vi "FPGANic-Tester.vi"() -> ()   [LabVIEW 2018]
uses:
  Source.Machine.Settings.ctl
  FPGANic.Events.ctl
  <vilib>/Field R&D Services/Logger/Private/Manager.vi
  <vilib>/FPGAPlugInAG/Dynamic/niLvFpga_Download_Dynamic.vi
  <vilib>/Utility/error.llb/Error Cluster From Error Code.vi
  <vilib>/rvi/errors/niLvFpgaAdjustHostInterfaceError.vi
  <vilib>/FPGAPlugInAG/Dynamic/niLvFpga_Run_Dynamic.vi
  FPGANic.Globals.vi
  <vilib>/FPGAPlugInAG/Dynamic/niLvFpga_Close_Dynamic.vi
  <vilib>/rvi/interface/nirviMethod/nirviMethod.xnode
  <vilib>/rvi/interface/nirviReadWriteControl/nirviReadWriteControl.xnode
  <vilib>/rvi/interface/nirviCloseFPGA/nirviCloseFPGA.xnode
  <vilib>/FPGAPlugInAG/Dynamic/niLvFpga_ReadFifo_Dynamic.vi
  <vilib>/rvi/errors/niLvFpgaMergeErrorWithErrorCode.vi
  <vilib>/FPGAPlugInAG/Dynamic/niLvFpga_WriteFifo_Dynamic.vi
  NiFpgaLv.dll
  <vilib>/rvi/interface/Simulation/niFpgaSimulationCallBeginRW.vi
  <vilib>/Field R&D Services/Logger/Logger.lvlib
panel:
  in  "Clear Debug FIFOS?":bool
  in  "Clear":bool
  in  "Read UART":bool
  in  "Tab Control":T1(tab)=enum."Configuration"
  in  "Ethernet II Params":T2={"Destination MAC"=[0, 2, 201, 85, 8, 68], "Source MAC"=[0, 1, 2, 3, 4, 5], "EtherType"=2048} {"Destination MAC" format="%.0x"; "Source MAC" format="%.02x"; "EtherType" format="%.0x"}
  in  "IPv4 Params":T3={"Destination IP"=[10, 0, 1, 100], "Source IP"=[10, 0, 1, 101], "Protocol"=17}
  in  "UDP Params":T4={"Source Port"=35312, "Destination Port"=35312, "Payload"="ABCD"}
  in  "MAC & IP":T5={"MAC Address"=[0, 1, 2, 3, 4, 5], "IP Address"=[10, 0, 1, 101]} {"MAC Address" format="%.0x"}
  out "Write Probe 2":u64[](array[numeric]) format="%.0x"
  out "Write Probe 1":u64[](array[numeric]) format="%.0x"
  out "Read Probe":u64[](array[numeric])=[11817445486661492224, 11817446517453291522, 11817445490022484036, 11817446517571077376, 11817445486650471966, 11817446518510649105, 11817445488139373056, 11817446517460230144, 11817445486661145833, 11817446517787656260, 11817445487417098240, 11817446519651434496, 11817445486644756480, 11817446517436909932, 11817445488513474924, 11817446519188976500, 11817445486735683427, 11817446519071309824, 11817445486669857024, 11817446517436872704, 11817445486712455169, 11817446519127149568, 11817445487441608960, 11817446517436872704, 11817445486741163008, 11817445692824123692, 11817726961621401602, 11817445490939658239, 11817446521731743746, 11817445490022484036, 11817446517571452929, 11817445486778910212, 11817446517436907522, 11817445490022484036, 11817446517604614500, 11817445486644690944, 11817446517436880915, 11817445488902144000, 11817446517436841984, 11817445486644690944, 11817446517436841984, 11817445486644690944, 11817445488835018955, 11817726961621401602, 11817445490939658239, 11817446521731743746, 11817445490022484036, 11817446517571452929, 11817445486778910212, 11817446517436907522, 11817445490022484036, 11817446517604614500, 11817445486644690944, 11817446517436895620, 11817445489682350080, 11817446517436841984, 11817445486644690944, 11817446517436841984, 11817445486644690944, 11817445488759354791, 11817726961621401602, 11817445490939658239, 11817446521731743746, 11817445490022484036, 11817446517571452929, 11817445486778910212, 11817446517436907522, 11817445490022484036, 11817446517604614500, 11817445486644690944, 11817446517436880915, 11817445488902144000, 11817446517436841984, 11817445486644690944, 11817446517436841984, 11817445486644690944, 11817445488835018955, 11817726961621401602, 11817445490939658239, 11817446521731743746, 11817445490022484036, 11817446517571452929, 11817445486778910212, 11817446517436907522, 11817445490022484036, 11817446517604614500, 11817445486644690944, 11817446517436878035, 11817445489493540864, 11817446517436841984, 11817445486644690944, 11817446517436841984, 11817445486644690944, 11817445489115705299, 11817726961621401602, 11817445490939658239, 11817446521731743746, 11817445490022484036, 11817446517571452929, 11817445486778910212, 11817446517436907522, 11817445490022484036, 11817446517604614500, 11817445486644690944, 11817446517436880915, 11817445488902144000, 11817446517436841984, 11817445486644690944, 11817446517436841984, 11817445486644690944, 11817445488835018955, 11817726961621401602, 11817445490939658239, 11817446521731743746, 11817445490022484036, 11817446517571452929, 11817445486778910212, 11817446517436907522, 11817445490022484036, 11817446517604614500, 11817445486644690944, 11817446517436878035, 11817445489493540864, 11817446517436841984, 11817445486644690944, 11817446517436841984, 11817445486644690944, 11817445489115705299, 11817726961621401602, 11817445490939658239, 11817446521731743746, 11817445490022484036, 11817446517571452929, 11817445486778910212, 11817446517436907522, 11817445490022484036, 11817446517604614500, 11817445486644690944, 11817446517436878035, 11817445489493540864, 11817446517436841984, 11817445486644690944, 11817446517436841984, 11817445486644690944, 11817445489115705299, 11817726961621401602, 11817445490939658239, 11817446521731743746, 11817445490022484036, 11817446517571452929, 11817445486778910212, 11817446517436907522, 11817445490022484036, 11817446517604614500, 11817445486644690944, 11817446517436880915, 11817445488902144000, 11817446517436841984, 11817445486644690944, 11817446517436841984, 11817445486644690944, 11817445488835018955, 11817726961621401602, 11817445486661492224, 11817446517453291522, 11817445490022484036, 11817446517571077376, 11817445486650474301, 11817446518510649105, 11817445487986346496, 11817446517460230144, 11817445486661145833, 11817446517787656260, 11817445487417098240, 11817446519651434496, 11817445486644756480, 11817446517436909932, 11817445488513474924, 11817446519188976500, 11817445486735683427, 11817446519071309824, 11817445486669857024, 11817446517436872704, 11817445486712455169, 11817446519127149568, 11817445487441608960, 11817446517436872704, 11817445486741163008, 11817445692824141017, 11817726961621401602, 11817445490939658239, 11817446521731743746, 11817445490022484036, 11817446517571452929, 11817445486778910212, 11817446517436907522, 11817445490022484036, 11817446517604614500, 11817445486644690944, 11817446517436878035, 11817445489493540864, 11817446517436841984, 11817445486644690944, 11817446517436841984, 11817445486644690944, 11817445489115705299, 11817726961621401602, 11817445490939658239, 11817446521731743746, 11817445490022484036, 11817446517571452929, 11817445486778910212, 11817446517436907522, 11817445490022484036, 11817446517604614500, 11817445486644690944, 11817446517436859339, 11817445486682636288, 11817446517436841984, 11817445486644690944, 11817446517436841984, 11817445486644690944, 11817445488555902218, 11817726961621401602, 11817445490939658239, 11817446521731743746, 11817445490022484036, 11817446517571452929, 11817445486778910212, 11817446517436907522, 11817445490022484036, 11817446517604614500, 11817445486644690944, 11817446517436859339, 11817445486682636288, 11817446517436841984, 11817445486644690944, 11817446517436841984, 11817445486644690944, 11817445488555902218, 11817726961621401602, 11817445490939658239, 11817446521731743746, 11817445490022484036, 11817446517571452929, 11817445486778910212, 11817446517436907522, 11817445490022484036, 11817446517604614500, 11817445486644690944, 11817446517436878035, 11817445489493540864, 11817446517436841984, 11817445486644690944, 11817446517436841984, 11817445486644690944, 11817445489115705299, 11817726961621401602, 11817445490939658239, 11817446521731743746, 11817445490022484036, 11817446517571452929, 11817445486778910212, 11817446517436907522, 11817445490022484036, 11817446517604614500, 11817445486644690944, 11817446517436878035, 11817445489493540864, 11817446517436841984, 11817445486644690944, 11817446517436841984, 11817445486644690944, 11817445489115705299, 11817726961621401602, 11817445490939658239, 11817446521731743746, 11817445490022484036, 11817446517571452929, 11817445486778910212, 11817446517436907522, 11817445490022484036, 11817446517604614500, 11817445486644690944, 11817446517436859339, 11817445486682636288, 11817446517436841984, 11817445486644690944, 11817446517436841984, 11817445486644690944, 11817445488555902218, 11817726961621401602, 11817445490939658239, 11817446521731743746, 11817445490022484036, 11817446517571452929, 11817445486778910212, 11817446517436907522, 11817445490022484036, 11817446517604614500, 11817445486644690944, 11817446517436859339, 11817445486682636288, 11817446517436841984, 11817445486644690944, 11817446517436841984, 11817445486644690944, 11817445488555902218, 11817726961621401602, 11817445490939658239, 11817446521731743746, 11817445490022484036, 11817446517571452929, 11817445486778910212, 11817446517436907522, 11817445490022484036, 11817446517604614500, 11817445486644690944, 11817446517436844075, 11817445488075145216, 11817446517436841984, 11817445486644690944, 11817446517436841984, 11817445486644690944, 11817445490337402917, 11817726961621401602, 11817445490939658239, 11817446521731743746, 11817445490022484036, 11817446517571452929, 11817445486778910212, 11817446517436907522, 11817445490022484036, 11817446517604614500, 11817445486644690944, 11817446517436859339, 11817445486682636288, 11817446517436841984, 11817445486644690944, 11817446517436841984, 11817445486644690944, 11817445488555902218, 11817726961621401602, 11817445490939658239, 11817446521731743746, 11817445490022484036, 11817446517571452929, 11817445486778910212, 11817446517436907522, 11817445490022484036, 11817446517604614500, 11817445486644690944, 11817446517436844075, 11817445488075145216, 11817446517436841984, 11817445486644690944, 11817446517436841984, 11817445486644690944, 11817445490337402917, 11817726961621401602, 11817445490939658239, 11817446521731743746, 11817445490022484036, 11817446517571452929, 11817445486778910212, 11817446517436907522, 11817445490022484036, 11817446517604614500, 11817445486644690944, 11817446517436859339, 11817445486682636288, 11817446517436841984, 11817445486644690944, 11817446517436841984, 11817445486644690944, 11817445488555902218, 11817726961621401602, 11817445490939658239, 11817446521731743746, 11817445490022484036, 11817446517571452929, 11817445486778910212, 11817446517436907522, 11817445490022484036, 11817446517604614500, 11817445486644690944, 11817446517436844075, 11817445488075145216, 11817446517436841984, 11817445486644690944, 11817446517436841984, 11817445486644690944, 11817445490337402917, 11817726961621401602, 11817445490939658239, 11817446521731743746, 11817445490022484036, 11817446517571452929, 11817445486778910212, 11817446517436907522, 11817445490022484036, 11817446517604614500, 11817445486644690944, 11817446517436844075, 11817445488075145216, 11817446517436841984, 11817445486644690944, 11817446517436841984, 11817445486644690944, 11817445490337402917, 11817726961621401602, 11817445490939658239, 11817446521731743746, 11817445490022484036, 11817446517571452929, 11817445486778910212, 11817446517436907522, 11817445490022484036, 11817446517604614500, 11817445486644690944, 11817446517436880915, 11817445488905814016, 11817446517436841984, 11817445486644690944, 11817446517436841984, 11817445486644690944, 11817445487441373583, 11817726961621401602, 11817445490939658239, 11817446521731743746, 11817445490022484036, 11817446517571452929, 11817445486778910212, 11817446517436907522, 11817445490022484036, 11817446517604614500, 11817445486644690944, 11817446517436844075, 11817445488075145216, 11817446517436841984, 11817445486644690944, 11817446517436841984, 11817445486644690944, 11817445490337402917, 11817726961621401602, 11817445490939658239, 11817446521731743746, 11817445490022484036, 11817446517571452929, 11817445486778910212, 11817446517436907522, 11817445490022484036, 11817446517604614500, 11817445486644690944, 11817446517436880915, 11817445488905814016, 11817446517436841984, 11817445486644690944, 11817446517436841984, 11817445486644690944, 11817445487441373583, 11817726961621401602, 11817445486661492224, 11817446517453291522, 11817445490022484036, 11817446517571077376, 11817445486650478677, 11817446518510649105, 11817445487699560960, 11817446517460230144, 11817445486661145833, 11817446517787656260, 11817445487417098240, 11817446519651434496, 11817445486644756480, 11817446517436909932, 11817445488513474924, 11817446519188976500, 11817445486735683427, 11817446519071309824, 11817445486669857024, 11817446517436872704, 11817445486712455169, 11817446519127149568, 11817445487441608960, 11817446517436872704, 11817445486741163008, 11817445692824141166, 11817726961621401602, 11817445490939658239, 11817446521731743746, 11817445490022484036, 11817446517571452929, 11817445486778910212, 11817446517436907522, 11817445490022484036, 11817446517604614500, 11817445486644690944, 11817446517436844075, 11817445488075145216, 11817446517436841984, 11817445486644690944, 11817446517436841984, 11817445486644690944, 11817445490337402917, 11817726961621401602, 11817445490939658239, 11817446521731743746, 11817445490022484036, 11817446517571452929, 11817445486778910212, 11817446517436907522, 11817445490022484036, 11817446517604614500, 11817445486644690944, 11817446517436880915, 11817445488905814016, 11817446517436841984, 11817445486644690944, 11817446517436841984, 11817445486644690944, 11817445487441373583, 11817726961621401602, 11817445490939658239, 11817446521731743746, 11817445490022484036, 11817446517571452929, 11817445486778910212, 11817446517436907522, 11817445490022484036, 11817446517604614500, 11817445486644690944, 11817446517436880915, 11817445488905814016, 11817446517436841984, 11817445486644690944, 11817446517436841984, 11817445486644690944, 11817445487441373583, 11817726961621401602, 11817445490939658239, 11817446521731743746, 11817445490022484036, 11817446517571452929, 11817445486778910212, 11817446517436907522, 11817445490022484036, 11817446517604614500, 11817445486644690944, 11817446517436859355, 11817445489065066496, 11817446517436841984, 11817445486644690944, 11817446517436841984, 11817445486644690944, 11817445488052856394, 11817726961621401602, 11817445490939658239, 11817446521731743746, 11817445490022484036, 11817446517571452929, 11817445486778910212, 11817446517436907522, 11817445490022484036, 11817446517604614500, 11817445486644690944, 11817446517436880915, 11817445488905814016, 11817446517436841984, 11817445486644690944, 11817446517436841984, 11817445486644690944, 11817445487441373583, 11817726961621401602, 11817445490939658239, 11817446521731743746, 11817445490022484036, 11817446517571452929, 11817445486778910212, 11817446517436907522, 11817445490022484036, 11817446517604614500, 11817445486644690944, 11817446517436859355, 11817445489065066496, 11817446517436841984, 11817445486644690944, 11817446517436841984, 11817445486644690944, 11817445488052856394, 11817726961621401602, 11817445490939658239, 11817446521731743746, 11817445490022484036, 11817446517571452929, 11817445486778910212, 11817446517436907522, 11817445490022484036, 11817446517604614500, 11817445486644690944, 11817446517436859355, 11817445489065066496, 11817446517436841984, 11817445486644690944, 11817446517436841984, 11817445486644690944, 11817445488052856394, 11817726961621401602, 11817445490939658239, 11817446521731743746, 11817445490022484036, 11817446517571452929, 11817445486778910212, 11817446517436907522, 11817445490022484036, 11817446517604614500, 11817445486644690944, 11817446517436880915, 11817445488905814016, 11817446517436841984, 11817445486644690944, 11817446517436841984, 11817445486644690944, 11817445487441373583, 11817726961621401602, 11817445490939658239, 11817446521731743746, 11817445490022484036, 11817446517571452929, 11817445486778910212, 11817446517436907522, 11817445490022484036, 11817446517604614500, 11817445486644690944, 11817446517436859355, 11817445489065066496, 11817446517436841984, 11817445486644690944, 11817446517436841984, 11817445486644690944, 11817445488052856394, 11817726961621401602, 11817445490939658239, 11817446521731743746, 11817445490022484036, 11817446517571452929, 11817445486778910212, 11817446517436907522, 11817445490022484036, 11817446517604614500, 11817445486644690944, 11817446517436878035, 11817445489492885504, 11817446517436841984, 11817445486644690944, 11817446517436841984, 11817445486644690944, 11817445490525715118, 11817726961621401602, 11817445490939658239, 11817446521731743746, 11817445490022484036, 11817446517571452929, 11817445486778910212, 11817446517436907522, 11817445490022484036, 11817446517604614500, 11817445486644690944, 11817446517436878035, 11817445489492885504, 11817446517436841984, 11817445486644690944, 11817446517436841984, 11817445486644690944, 11817445490525715118, 11817726961621401602, 11817445490939658239, 11817446521731743746, 11817445490022484036, 11817446517571452929, 11817445486778910212, 11817446517436907522, 11817445490022484036, 11817446517604614500, 11817445486644690944, 11817446517436859355, 11817445489065066496, 11817446517436841984, 11817445486644690944, 11817446517436841984, 11817445486644690944, 11817445488052856394, 11817726961621401602, 11817445490939658239, 11817446521731743746, 11817445490022484036, 11817446517571452929, 11817445486778910212, 11817446517436907522, 11817445490022484036, 11817446517604614500, 11817445486644690944, 11817446517436859355, 11817445489065066496, 11817446517436841984, 11817445486644690944, 11817446517436841984, 11817445486644690944, 11817445488052856394, 11817726961621401602, 11817445490939658239, 11817446521731743746, 11817445490022484036, 11817446517571452929, 11817445486778910212, 11817446517436907522, 11817445490022484036, 11817446517604614500, 11817445486644690944, 11817446517436878035, 11817445489492885504, 11817446517436841984, 11817445486644690944, 11817446517436841984, 11817445486644690944, 11817445490525715118, 11817726961621401602, 11817445490939658239, 11817446521731743746, 11817445490022484036, 11817446517571452929, 11817445486778910212, 11817446517436907522, 11817445490022484036, 11817446517604614500, 11817445486644690944, 11817446517436878035, 11817445489492885504, 11817446517436841984, 11817445486644690944, 11817446517436841984, 11817445486644690944, 11817445490525715118, 11817726961621401602, 11817445490939658239, 11817446521731743746, 11817445490022484036, 11817446517571452929, 11817445486778910212, 11817446517436907522, 11817445490022484036, 11817446517604614500, 11817445486644690944, 11817446517436858915, 11817445487695495168, 11817446517436841984, 11817445486644690944, 11817446517436841984, 11817445486644690944, 11817445489806603878, 11817726961621401602, 11817445490939658239, 11817446521731743746, 11817445490022484036, 11817446517571452929, 11817445486778910212, 11817446517436907522, 11817445490022484036, 11817446517604614500, 11817445486644690944, 11817446517436878035, 11817445489492885504, 11817446517436841984, 11817445486644690944, 11817446517436841984, 11817445486644690944, 11817445490525715118, 11817726961621401602, 11817445490939658239, 11817446521731743746, 11817445490022484036, 11817446517571452929, 11817445486778910212, 11817446517436907522, 11817445490022484036, 11817446517604614500, 11817445486644690944, 11817446517436858915, 11817445487695495168, 11817446517436841984, 11817445486644690944, 11817446517436841984, 11817445486644690944, 11817445489806603878, 11817726961621401602, 11817445486661492224, 11817446517453291522, 11817445490022484036, 11817446517571077376, 11817445486649761975, 11817446518510649105, 11817445487425423872, 11817446517460230144, 11817445486661145833, 11817446517787656249, 11817445488492281856, 11817446517436841985, 11817445486644690945, 11817446517436844396, 11817445488513474924, 11817446519188976500, 11817445486735683427, 11817446519071309824, 11817445490922881472, 11817446517638168832, 11817445486661468160, 11817446519450108938, 11817445486644782091, 11817445453811713277, 11817726961621401602, 11817445486661492224, 11817446517453291522, 11817445490022484036, 11817446517571077376, 11817445486649762087, 11817446518510649105, 11817445487418083840, 11817446517460230144, 11817445486661145833, 11817446517787656249, 11817445488492281856, 11817446517436841985, 11817445486644690945, 11817446517436844396, 11817445488513474924, 11817446519188976500, 11817445486735683427, 11817446519071309824, 11817445490922881472, 11817446517638168832, 11817445486661468160, 11817446519450108938, 11817445486644782266, 11817445452738132989, 11817726961621401602, 11817445490939658239, 11817446521731743746, 11817445490022484036, 11817446517571452929, 11817445486778910212, 11817446517436907522, 11817445490022484036, 11817446517604614500, 11817445486644690944, 11817446517436878035, 11817445489492885504, 11817446517436841984, 11817445486644690944, 11817446517436841984, 11817445486644690944, 11817445490525715118, 11817726961621401602, 11817445490939658239, 11817446521731743746, 11817445490022484036, 11817446517571452929, 11817445486778910212, 11817446517436907522, 11817445490022484036, 11817446517604614500, 11817445486644690944, 11817446517436858915, 11817445487695495168, 11817446517436841984, 11817445486644690944, 11817446517436841984, 11817445486644690944, 11817445489806603878, 11817726961621401602, 11817445486661492224, 11817446517453291522, 11817445490022484036, 11817446517571077376, 11817445486649762234, 11817446518510649105, 11817445487408450048, 11817446517460230144, 11817445486661145833, 11817446517787656249, 11817445488492281856, 11817446517436841985, 11817445486644690945, 11817446517436844396, 11817445488513474924, 11817446519188976500, 11817445486735683427, 11817446519071309824, 11817445490922881472, 11817446517638168832, 11817445486661468160, 11817446519450108938, 11817445486644782315, 11817445454750429437, 11817726961621401602, 11817445486661492224, 11817446517453291522, 11817445490022484036, 11817446517571077376, 11817445486652908126, 11817446518510649105, 11817445487394556416, 11817446517460230144, 11817445486661145833, 11817446517787656297, 11817445488489922560, 11817446519651434496, 11817445486644822016, 11817446517436909932, 11817445488513474924, 11817446519188976500, 11817445486735683427, 11817446519071309824, 11817445486669857024, 11817446517436872704, 11817445486712455169, 11817446519114772784, 11817445487450075393, 11817446518242292016, 11817445486769040941, 11817446519070811250, 11817445486718186096, 11817446519064231948, 11817445488792240128, 11817446517444706306, 11817445489866752012, 11817446517439954945, 11817445486644691064, 11817446517437218828, 11817445486644773000, 11817445453377722877, 11817726961621401602, 11817445486661492224, 11817446517453291522, 11817445490022484036, 11817446517571077376, 11817445486651073205, 11817446518510649105, 11817445487390689792, 11817446517460230144, 11817445486661145833, 11817446517787656269, 11817445487799631872, 11817446517436841985, 11817445486644690945, 11817446517436842801, 11817445487453143345, 11817446517456765489, 11817445487450483054, 11817446518198199396, 11817445488557580658, 11817446519322247168, 11817445490922881472, 11817446517638171648, 11817445486661468160, 11817446519450112008, 11817445488463539829, 11817446519453069873, 11817445486735683427, 11817445969315496190, 11817726961621401602, 11817445486661492224, 11817446517453291522, 11817445490022484036, 11817446517571077376, 11817445486651073370, 11817446518510649105, 11817445487379876352, 11817446517460230144, 11817445486661145833, 11817446517787656269, 11817445487799631872, 11817446517436841985, 11817445486644690945, 11817446517436842801, 11817445487453143345, 11817446517456765489, 11817445487450483054, 11817446518198199396, 11817445488557580658, 11817446519322247168, 11817445490922881472, 11817446517638171648, 11817445486661468160, 11817446519450112008, 11817445488463539829, 11817446519453069873, 11817445486735683427, 11817445969315496167, 11817726961621401602, 11817445486661492224, 11817446517453291522, 11817445490022484036, 11817446517571077376, 11817445486651073405, 11817446518510649105, 11817445487377582592, 11817446517460230144, 11817445486661145833, 11817446517787656269, 11817445487799631872, 11817446517436841985, 11817445486644690945, 11817446517436842801, 11817445487453143345, 11817446517456765489, 11817445487450483054, 11817446518198199396, 11817445488557580658, 11817446519322247168, 11817445490922881472, 11817446517638171648, 11817445486661468160, 11817446519450112008, 11817445488463539829, 11817446519453069873, 11817445486735683427, 11817445969315495936, 11817726961621401602, 11817445486661492224, 11817446517453291522, 11817445490022484036, 11817446517571077376, 11817445486650680210, 11817446518510649105, 11817445487376599552, 11817446517460230144, 11817445486661145833, 11817446517787656263, 11817445490086379520, 11817446519651434496, 11817445486644756480, 11817446517436842801, 11817445487453143345, 11817446517456765489, 11817445487450483054, 11817446518198199396, 11817445488557580658, 11817446519322247168, 11817445486854406400, 11817446517436872704, 11817445486913678441, 11817446519290034221, 11817445487486764396, 11817446519305625964, 11817445486650109318, 11817445428830209799, 11817726961621401602, 11817445486661492224, 11817446517453291522, 11817445490022484036, 11817446517571077376, 11817445486650483777, 11817446518510649105, 11817445487365327360, 11817446517460230144, 11817445486661145833, 11817446517787656260, 11817445487417098240, 11817446519651434496, 11817445486644756480, 11817446517436909932, 11817445488513474924, 11817446519188976500, 11817445486735683427, 11817446519071309824, 11817445486669857024, 11817446517436872704, 11817445486712455169, 11817446519127149568, 11817445487441608960, 11817446517436872704, 11817445486741163008, 11817445692824112747, 11817726961621401602, 11817445486661492224, 11817446517453291522, 11817445490022484036, 11817446517571077376, 11817445486650674912, 11817446518510649105, 11817445487723809280, 11817446517460230144, 11817445486661145833, 11817446517787656263, 11817445490086379520, 11817446519651434496, 11817445486644756480, 11817446517436842801, 11817445487453143345, 11817446517456765489, 11817445487450483054, 11817446518198199396, 11817445488557580658, 11817446519322247168, 11817445486854406400, 11817446517436872704, 11817445486913678441, 11817446519290034221, 11817445487486764396, 11817446519305625964, 11817445486652761861, 11817445427538364167, 11817726961621401602, 11817445490939658239, 11817446521731743746, 11817445490022484036, 11817446517571452929, 11817445486778910212, 11817446517436907522, 11817445490022484036, 11817446517604614500, 11817445486644690944, 11817446517436878035, 11817445489492885504, 11817446517436841984, 11817445486644690944, 11817446517436841984, 11817445486644690944, 11817445490525715118, 11817726961621401602, 11817445490939658239, 11817446521731743746, 11817445490022484036, 11817446517571452929, 11817445486778910212, 11817446517436907522, 11817445490022484036, 11817446517604614500, 11817445486644690944, 11817446517436844075, 11817445488075145216, 11817446517436841984, 11817445486644690944, 11817446517436841984, 11817445486644690944, 11817445490337402917, 11817726961621401602, 11817445486661492224, 11817446517453291522, 11817445490022484036, 11817446517571077376, 11817445486650478551, 11817446518510649105, 11817445487707818496, 11817446517460230144, 11817445486661145833, 11817446517787656260, 11817445487417098240, 11817446519651434496, 11817445486644756480, 11817446517436909932, 11817445488513474924, 11817446519188976500, 11817445486735683427, 11817446519071309824, 11817445486669857024, 11817446517436872704, 11817445486712455169, 11817446519127149568, 11817445487441608960, 11817446517436872704, 11817445486741163008, 11817445692824104959, 11817726961621401602, 11817445490939658239, 11817446521731743746, 11817445490022484036, 11817446517571452929, 11817445486778910212, 11817446517436907522, 11817445490022484036, 11817446517604614500, 11817445486644690944, 11817446517436844075, 11817445488075145216, 11817446517436841984, 11817445486644690944, 11817446517436841984, 11817445486644690944, 11817445490337402917, 11817726961621401602, 11817445490939658239, 11817446521731743746, 11817445490022484036, 11817446517571452929, 11817445486778910212, 11817446517436907522, 11817445490022484036, 11817446517604614500, 11817445486644690944, 11817446517436880915, 11817445488905814016, 11817446517436841984, 11817445486644690944, 11817446517436841984, 11817445486644690944, 11817445487441373583, 11817726961621401602, 11817445486661492224, 11817446517453291522, 11817445490022484036, 11817446517571077376, 11817445486650675876, 11817446518510649105, 11817445487660632576, 11817446517460230144, 11817445486661145833, 11817446517787656263, 11817445490086379520, 11817446519651434496, 11817445486644756480, 11817446517436842801, 11817445487453143345, 11817446517456765489, 11817445487450483054, 11817446518198199396, 11817445488557580658, 11817446519322247168, 11817445486854406400, 11817446517436872704, 11817445486913678441, 11817446519290034221, 11817445487486764396, 11817446519305625964, 11817445486655633830, 11817445428595328775, 11817726961621401602, 11817445490939658239, 11817446521731743746, 11817445490022484036, 11817446517571452929, 11817445486778910212, 11817446517436907522, 11817445490022484036, 11817446517604614500, 11817445486644690944, 11817446517436880915, 11817445488905814016, 11817446517436841984, 11817445486644690944, 11817446517436841984, 11817445486644690944, 11817445487441373583, 11817726961621401602, 11817445490939658239, 11817446521731743746, 11817445490022484036, 11817446517571452929, 11817445486778910212, 11817446517436907522, 11817445490022484036, 11817446517604614500, 11817445486644690944, 11817446517436844075, 11817445488075145216, 11817446517436841984, 11817445486644690944, 11817446517436841984, 11817445486644690944, 11817445490337402917, 11817726961621401602, 11817445490939658239, 11817446521731743746, 11817445490022484036, 11817446517571452929, 11817445486778910212, 11817446517436907522, 11817445490022484036, 11817446517604614500, 11817445486644690944, 11817446517436844075, 11817445488075145216, 11817446517436841984, 11817445486644690944, 11817446517436841984, 11817445486644690944, 11817445490337402917, 11817726961621401602, 11817445490939658239, 11817446521731743746, 11817445490022484036, 11817446517571452929, 11817445486778910212, 11817446517436907522, 11817445490022484036, 11817446517604614500, 11817445486644690944, 11817446517436880915, 11817445488905814016, 11817446517436841984, 11817445486644690944, 11817446517436841984, 11817445486644690944, 11817445487441373583, 11817726961621401602, 11817445490939658239, 11817446521731743746, 11817445490022484036, 11817446517571452929, 11817445486778910212, 11817446517436907522, 11817445490022484036, 11817446517604614500, 11817445486644690944, 11817446517436880915, 11817445488905814016, 11817446517436841984, 11817445486644690944, 11817446517436841984, 11817445486644690944, 11817445487441373583, 11817726961621401602, 11817445490939658239, 11817446521731743746, 11817445490022484036, 11817446517571452929, 11817445486778910212, 11817446517436907522, 11817445490022484036, 11817446517604614500, 11817445486644690944, 11817446517436878035, 11817445489493540864, 11817446517436841984, 11817445486644690944, 11817446517436841984, 11817445486644690944, 11817445489115705299, 11817726961621401602, 11817445486661492224, 11817446517453291522, 11817445490022484036, 11817446517571077376, 11817445486650481225, 11817446518510649105, 11817445487532575232, 11817446517460230144, 11817445486661145833, 11817446517787656260, 11817445487417098240, 11817446519651434496, 11817445486644756480, 11817446517436909932, 11817445488513474924, 11817446519188976500, 11817445486735683427, 11817446519071309824, 11817445486669857024, 11817446517436872704, 11817445486712455169, 11817446519127149568, 11817445487441608960, 11817446517436872704, 11817445486741163008, 11817445692824103053, 11817726961621401602, 11817445490939658239, 11817446521731743746, 11817445490022484036, 11817446517571452929, 11817445486778910212, 11817446517436907522, 11817445490022484036, 11817446517604614500, 11817445486644690944, 11817446517436880915, 11817445488905814016, 11817446517436841984, 11817445486644690944, 11817446517436841984, 11817445486644690944, 11817445487441373583, 11817726961621401602, 11817445490939658239, 11817446521731743746, 11817445490022484036, 11817446517571452929, 11817445486778910212, 11817446517436907522, 11817445490022484036, 11817446517604614500, 11817445486644690944, 11817446517436878035, 11817445489493540864, 11817446517436841984, 11817445486644690944, 11817446517436841984, 11817445486644690944, 11817445489115705299, 11817726961621401602, 11817445490939658239, 11817446521731743746, 11817445490022484036, 11817446517571452929, 11817445486778910212, 11817446517436907522, 11817445490022484036, 11817446517604614500, 11817445486644690944, 11817446517436878035, 11817445489493540864, 11817446517436841984, 11817445486644690944, 11817446517436841984, 11817445486644690944, 11817445489115705299, 11817726961621401602, 11817445490939658239, 11817446521731743746, 11817445490022484036, 11817446517571452929, 11817445486778910212, 11817446517436907522, 11817445490022484036, 11817446517604614500, 11817445486644690944, 11817446517436880915, 11817445488905814016, 11817446517436841984, 11817445486644690944, 11817446517436841984, 11817445486644690944, 11817445487441373583, 11817726961621401602, 11817445490939658239, 11817446521731743746, 11817445490022484036, 11817446517571452929, 11817445486778910212, 11817446517436907522, 11817445490022484036, 11817446517604614500, 11817445486644690944, 11817446517436878035, 11817445489493540864, 11817446517436841984, 11817445486644690944, 11817446517436841984, 11817445486644690944, 11817445489115705299, 11817726961621401602, 11817445490939658239, 11817446521731743746, 11817445490022484036, 11817446517571452929, 11817445486778910212, 11817446517436907522, 11817445490022484036, 11817446517604614500, 11817445486644690944, 11817446517436889485, 11817445489429577728, 11817446517436841984, 11817445486644690944, 11817446517436841984, 11817445486644690944, 11817445488947655731, 11817726961621401602, 11817445490939658239, 11817446521731743746, 11817445490022484036, 11817446517571452929, 11817445486778910212, 11817446517436907522, 11817445490022484036, 11817446517604614500, 11817445486644690944, 11817446517436889485, 11817445489429577728, 11817446517436841984, 11817445486644690944, 11817446517436841984, 11817445486644690944, 11817445488947655731, 11817726961621401602, 11817445490939658239, 11817446521731743746, 11817445490022484036, 11817446517571452929, 11817445486778910212, 11817446517436907522, 11817445490022484036, 11817446517604614500, 11817445486644690944, 11817446517436878035, 11817445489493540864, 11817446517436841984, 11817445486644690944, 11817446517436841984, 11817445486644690944, 11817445489115705299, 11817726961621401602, 11817445490939658239, 11817446521731743746, 11817445490022484036, 11817446517571452929, 11817445486778910212, 11817446517436907522, 11817445490022484036, 11817446517604614500, 11817445486644690944, 11817446517436878035, 11817445489493540864, 11817446517436841984, 11817445486644690944, 11817446517436841984, 11817445486644690944, 11817445489115705299, 11817726961621401602, 11817445490939658239, 11817446521731743746, 11817445490022484036, 11817446517571452929, 11817445486778910212, 11817446517436907522, 11817445490022484036, 11817446517604614500, 11817445486644690944, 11817446517436889485, 11817445489429577728, 11817446517436841984, 11817445486644690944, 11817446517436841984, 11817445486644690944, 11817445488947655731, 11817726961621401602, 11817445490939658239, 11817446521731743746, 11817445490022484036, 11817446517571452929, 11817445486778910212, 11817446517436907522, 11817445490022484036, 11817446517604614500, 11817445486644690944, 11817446517436889485, 11817445489429577728, 11817446517436841984, 11817445486644690944, 11817446517436841984, 11817445486644690944, 11817445488947655731, 11817726961621401602, 11817445490939658239, 11817446521731743746, 11817445490022484036, 11817446517571452929, 11817445486778910212, 11817446517436907522, 11817445490022484036, 11817446517604614500, 11817445486644690944, 11817446517436895620, 11817445489682350080, 11817446517436841984, 11817445486644690944, 11817446517436841984, 11817445486644690944, 11817445488759354791, 11817726961621401602, 11817445490939658239, 11817446521731743746, 11817445490022484036, 11817446517571452929, 11817445486778910212, 11817446517436907522, 11817445490022484036, 11817446517604614500, 11817445486644690944, 11817446517436889485, 11817445489429577728, 11817446517436841984, 11817445486644690944, 11817446517436841984, 11817445486644690944, 11817445488947655731, 11817726961621401602, 11817445490939658239, 11817446521731743746, 11817445490022484036, 11817446517571452929, 11817445486778910212, 11817446517436907522, 11817445490022484036, 11817446517604614500, 11817445486644690944, 11817446517436895620, 11817445489682350080, 11817446517436841984, 11817445486644690944, 11817446517436841984, 11817445486644690944, 11817445488759354791, 11817726961621401602, 11817445490939658239, 11817446521731743746, 11817445490022484036, 11817446517571452929, 11817445486778910212, 11817446517436907522, 11817445490022484036, 11817446517604614500, 11817445486644690944, 11817446517436895620, 11817445489682350080, 11817446517436841984, 11817445486644690944, 11817446517436841984, 11817445486644690944, 11817445488759354791, 11817726961621401602, 11817445490939658239, 11817446521731743746, 11817445490022484036, 11817446517571452929, 11817445486778910212, 11817446517436907522, 11817445490022484036, 11817446517604614500, 11817445486644690944, 11817446517436889485, 11817445489429577728, 11817446517436841984, 11817445486644690944, 11817446517436841984, 11817445486644690944, 11817445488947655731, 11817726961621401602, 11817445486661492224, 11817446517453291522, 11817445490022484036, 11817446517571077376, 11817445486650485803, 11817446518510649105, 11817445487232551424, 11817446517460230144, 11817445486661145833, 11817446517787656260, 11817445487417098240, 11817446519651434496, 11817445486644756480, 11817446517436909932, 11817445488513474924, 11817446519188976500, 11817445486735683427, 11817446519071309824, 11817445486669857024, 11817446517436872704, 11817445486712455169, 11817446519127149568, 11817445487441608960, 11817446517436872704, 11817445486741163008, 11817445692824156020, 11817726961621401602, 11817445490939658239, 11817446521731743746, 11817445490022484036, 11817446517571452929, 11817445486778910212, 11817446517436907522, 11817445490022484036, 11817446517604614500, 11817445486644690944, 11817446517436895620, 11817445489682350080, 11817446517436841984, 11817445486644690944, 11817446517436841984, 11817445486644690944, 11817445488759354791, 11817726961621401602, 11817445490939658239, 11817446521731743746, 11817445490022484036, 11817446517571452929, 11817445486778910212, 11817446517436907522, 11817445490022484036, 11817446517604614500, 11817445486644690944, 11817446517436880915, 11817445488902144000, 11817446517436841984, 11817445486644690944, 11817446517436841984, 11817445486644690944, 11817445488835018955, 11817726961621401602, 11817445490939658239, 11817446521731743746, 11817445490022484036, 11817446517571452929, 11817445486778910212, 11817446517436907522, 11817445490022484036, 11817446517604614500, 11817445486644690944, 11817446517436880915, 11817445488902144000, 11817446517436841984, 11817445486644690944, 11817446517436841984, 11817445486644690944, 11817445488835018955, 11817726961621401602, 11817445490939658239, 11817446521731743746, 11817445490022484036, 11817446517571452929, 11817445486778910212, 11817446517436907522, 11817445490022484036, 11817446517604614500, 11817445486644690944, 11817446517436895620, 11817445489682350080, 11817446517436841984, 11817445486644690944, 11817446517436841984, 11817445486644690944, 11817445488759354791, 11817726961621401602, 11817445490939658239, 11817446521731743746, 11817445490022484036, 11817446517571452929, 11817445486778910212, 11817446517436907522, 11817445490022484036, 11817446517604614500, 11817445486644690944, 11817446517436895620, 11817445489682350080, 11817446517436841984, 11817445486644690944, 11817446517436841984, 11817445486644690944, 11817445488759354791, 11817726961621401602, 11817445490939658239, 11817446521731743746, 11817445490022484036, 11817446517571452929, 11817445486778910212, 11817446517436907522, 11817445490022484036, 11817446517604614500, 11817445486644690944, 11817446517436880915, 11817445488902144000, 11817446517436841984, 11817445486644690944, 11817446517436841984, 11817445486644690944, 11817445488835018955, 11817726961621401602, 11817445490939658239, 11817446521731743746, 11817445490022484036, 11817446517571452929, 11817445486778910212, 11817446517436907522, 11817445490022484036, 11817446517604614500, 11817445486644690944, 11817446517436880915, 11817445488902144000, 11817446517436841984, 11817445486644690944, 11817446517436841984, 11817445486644690944, 11817445488835018955, 11817726961621401602, 11817445490939658239, 11817446521731743746, 11817445490022484036, 11817446517571452929, 11817445486778910212, 11817446517436907522, 11817445490022484036, 11817446517604614500, 11817445486644690944, 11817446517436859355, 11817445489065066496, 11817446517436841984, 11817445486644690944, 11817446517436841984, 11817445486644690944, 11817445488052856394, 11817726961621401602, 11817445490939658239, 11817446521731743746, 11817445490022484036, 11817446517571452929, 11817445486778910212, 11817446517436907522, 11817445490022484036, 11817446517604614500, 11817445486644690944, 11817446517436859355, 11817445489065066496, 11817446517436841984, 11817445486644690944, 11817446517436841984, 11817445486644690944, 11817445488052856394, 11817726961621401602, 11817445490939658239, 11817446521731743746, 11817445490022484036, 11817446517571452929, 11817445486778910212, 11817446517436907522, 11817445490022484036, 11817446517604614500, 11817445486644690944, 11817446517436880915, 11817445488902144000, 11817446517436841984, 11817445486644690944, 11817446517436841984, 11817445486644690944, 11817445488835018955, 11817726961621401602, 11817445490939658239, 11817446521731743746, 11817445490022484036, 11817446517571452929, 11817445486778910212, 11817446517436907522, 11817445490022484036, 11817446517604614500, 11817445486644690944, 11817446517436880915, 11817445488902144000, 11817446517436841984, 11817445486644690944, 11817446517436841984, 11817445486644690944, 11817445488835018955, 11817726961621401602, 11817445490939658239, 11817446521731743746, 11817445490022484036, 11817446517571452929, 11817445486778910212, 11817446517436907522, 11817445490022484036, 11817446517604614500, 11817445486644690944, 11817446517436859355, 11817445489065066496, 11817446517436841984, 11817445486644690944, 11817446517436841984, 11817445486644690944, 11817445488052856394, 11817726961621401602, 11817445490939658239, 11817446521731743746, 11817445490022484036, 11817446517571452929, 11817445486778910212, 11817446517436907522, 11817445490022484036, 11817446517604614500, 11817445486644690944, 11817446517436859355, 11817445489065066496, 11817446517436841984, 11817445486644690944, 11817446517436841984, 11817445486644690944, 11817445488052856394, 11817726961621401602, 11817445490939658239, 11817446521731743746, 11817445490022484036, 11817446517571452929, 11817445486778910212, 11817446517436907522, 11817445490022484036, 11817446517604614500, 11817445486644690944, 11817446517436859355, 11817445489065066496, 11817446517436841984, 11817445486644690944, 11817446517436841984, 11817445486644690944, 11817445488052856394, 11817726961621401602, 11817445490939658239, 11817446521731743746, 11817445490022484036, 11817446517571452929, 11817445486778910212, 11817446517436907522, 11817445490022484036, 11817446517604614500, 11817445486644690944, 11817446517436859355, 11817445489065066496, 11817446517436841984, 11817445486644690944, 11817446517436841984, 11817445486644690944, 11817445488052856394, 11817726961621401602, 11817445486661492224, 11817446517453291522, 11817445490022484036, 11817446517571077376, 11817445486650497716, 11817446518510649105, 11817445490746722816, 11817446517460230144, 11817445486661145833, 11817446517787656260, 11817445487417098240, 11817446519651434496, 11817445486644756480, 11817446517436909932, 11817445488513474924, 11817446519188976500, 11817445486735683427, 11817446519071309824, 11817445486669857024, 11817446517436872704, 11817445486712455169, 11817446519127149568, 11817445487441608960, 11817446517436872704, 11817445486741163008, 11817445692824105340, 11817726961621401602, 11817445490939658239, 11817446521731743746, 11817445490022484036, 11817446517571452929, 11817445486778910212, 11817446517436907522, 11817445490022484036, 11817446517604614500, 11817445486644690944, 11817446517436844544, 11817445486668087296, 11817446517436841984, 11817445486644690944, 11817446517436841984, 11817445486644690944, 11817445488739790818, 11817726961621401602, 11817445490939658239, 11817446521731743746, 11817445490022484036, 11817446517571452929, 11817445486778910212, 11817446517436907522, 11817445490022484036, 11817446517604614500, 11817445486644690944, 11817446517436844544, 11817445486668087296, 11817446517436841984, 11817445486644690944, 11817446517436841984, 11817445486644690944, 11817445488739790818, 11817726961621401602, 11817445490939658239, 11817446521731743746, 11817445490022484036, 11817446517571452929, 11817445486778910212, 11817446517436907522, 11817445490022484036, 11817446517604614500, 11817445486644690944, 11817446517436844544, 11817445486668087296, 11817446517436841984, 11817445486644690944, 11817446517436841984, 11817445486644690944, 11817445488739790818, 11817726961621401602] format="%.0x"
  out "Debug FIFO 2":u32[](array[numeric])=[1, 3, 43680, 1, 3, 43680] format="%.0x"
  out "Debug FIFO 1":u32[](array[numeric]) format="%.0x"
  out "Response":u8[](array[numeric]) format="%.0x"
  out "In Payload":u8[](array[numeric]) format="%.0x"
  in  "Read Polling?":bool
  out "Bitfile Downloaded":bool
  in  "lvbitx file":path=path "C:/Users/John/Desktop/FPGATester/fpga_nic.lvbitx"
  in  "AXI_STR_RXD_3_tkeep":u8=15
  out "GPIO #1 out":u32 format="%.0x"
  in  "GPIO #2 in":u32=6 format="%.0x"
  in  "GPIO #1 in":u32=6 format="%.0x"
  out "GPIO #2 out":u32 format="%.0x"
  out "sPort0_Power_Good":bool
  out "signal_detect_Port0":bool
  out "aBlockLockPort0":bool
  out "UART Receive":string
  out "FPGA Ready":bool
  in  "Start":bool
  in  "Device address":string="RIO0"
  in  "UART Polling?":bool=TRUE
  in  "Read/Write GPIO":bool
  out "error out":errorcluster
  out "Status":string
  in  "error in":errorcluster
  in  "Exit":bool
  in  "Transmit Packet":bool
  in  "Read Packet":bool
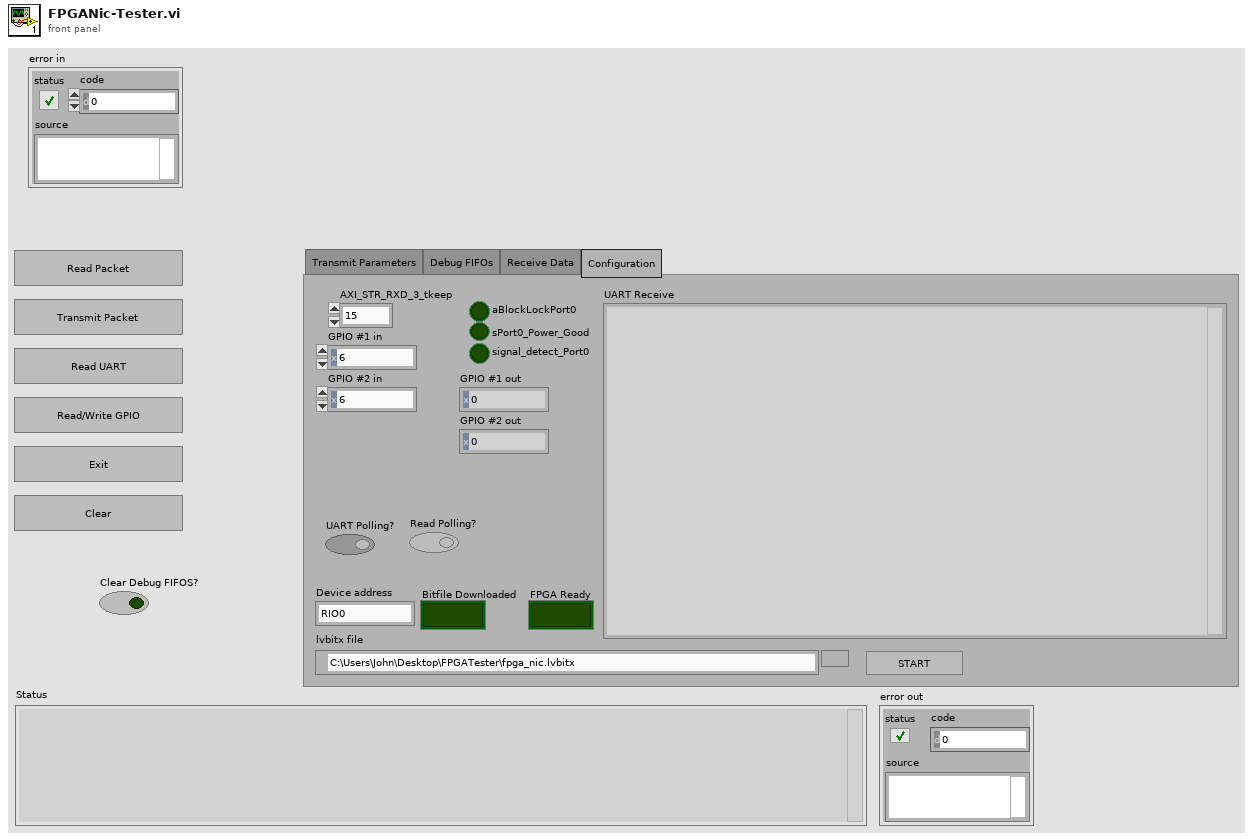
[diagram p1: front panel]
types:
  T1 = enum32{"Transmit Parameters", "Debug FIFOs", "Receive Data", "Configuration"}
  T2 = cluster{"Destination MAC":u8[], "Source MAC":u8[], "EtherType":u16}
  T3 = cluster{"Destination IP":u8[], "Source IP":u8[], "Protocol":u8}
  T4 = cluster{"Source Port":u16, "Destination Port":u16, "Payload":string}
  T5 = typedef "Source.Machine.Settings.ctl" = cluster{"MAC Address":u8[], "IP Address":u8[]}
  T6 = typedef "FPGANic.Events.ctl" = enum16{"Open FPGA", "Close FPGA", "Reset UI", "Read Packet", "Transmit Packet", "Read UART", "Read Probes", "Read/Write GPIO"}
  T7 = cluster{"Read Probe":u64[], "Write Probe 1":u64[], "Write Probe 2":u64[], "Debug FIFO 1":u32[], "Debug FIFO 2":u32[]}
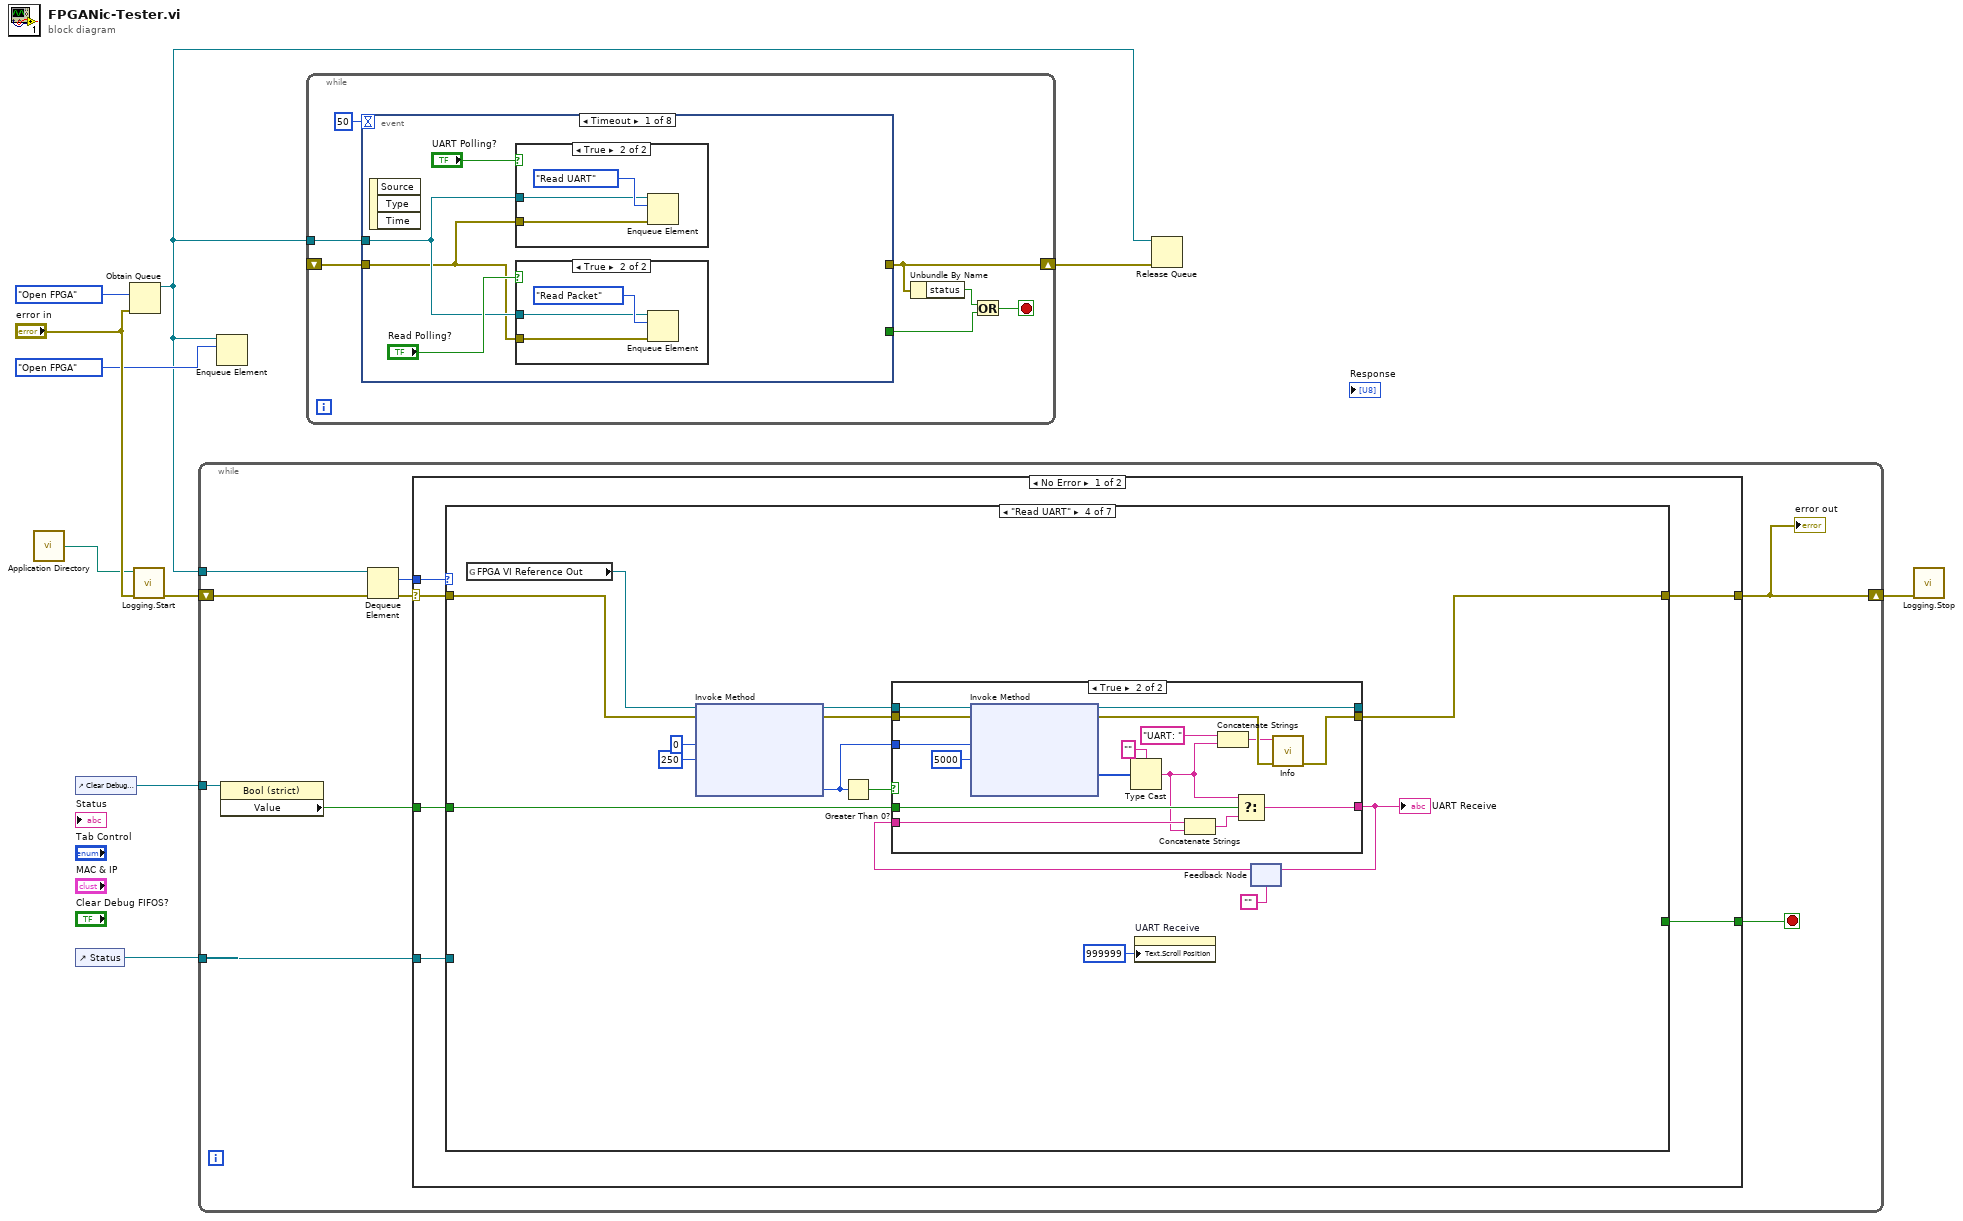
[diagram p0: block diagram]
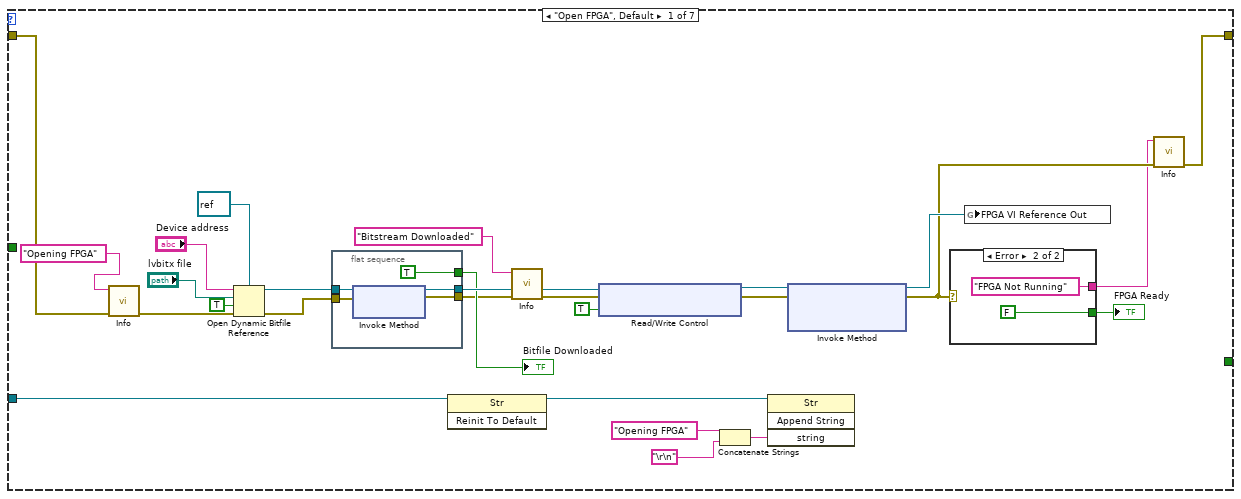
[diagram p2: hidden frame]
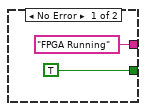
[diagram p3: hidden frame]
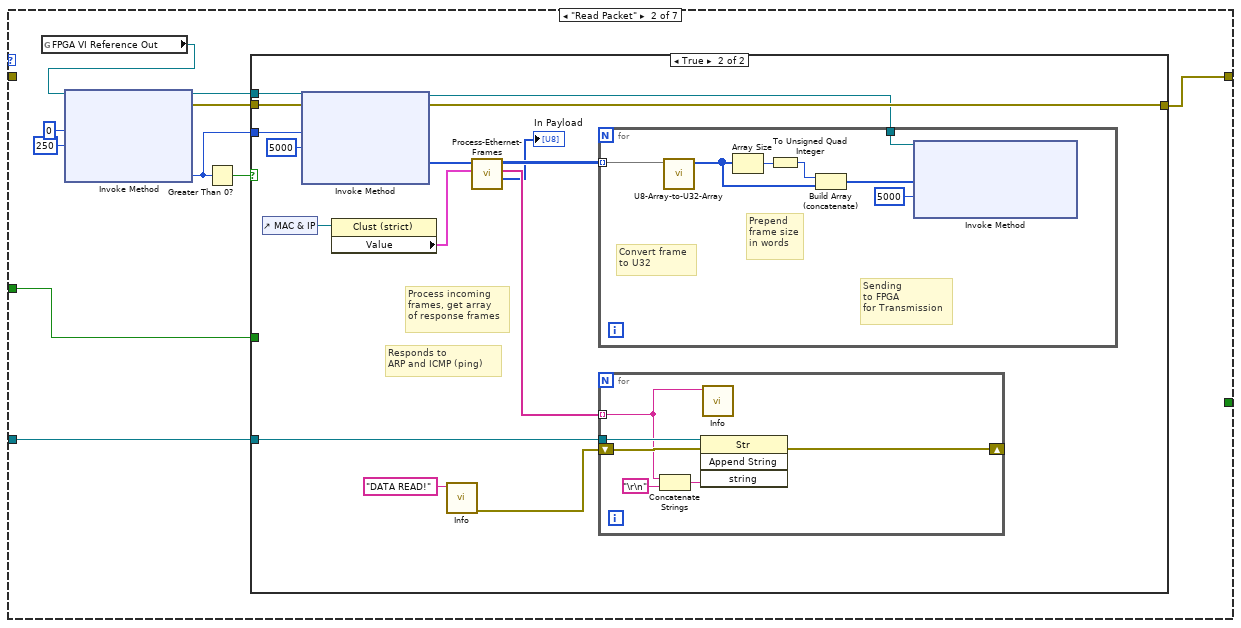
[diagram p4: hidden frame]
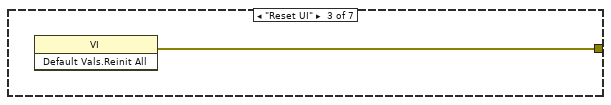
[diagram p6: hidden frame]
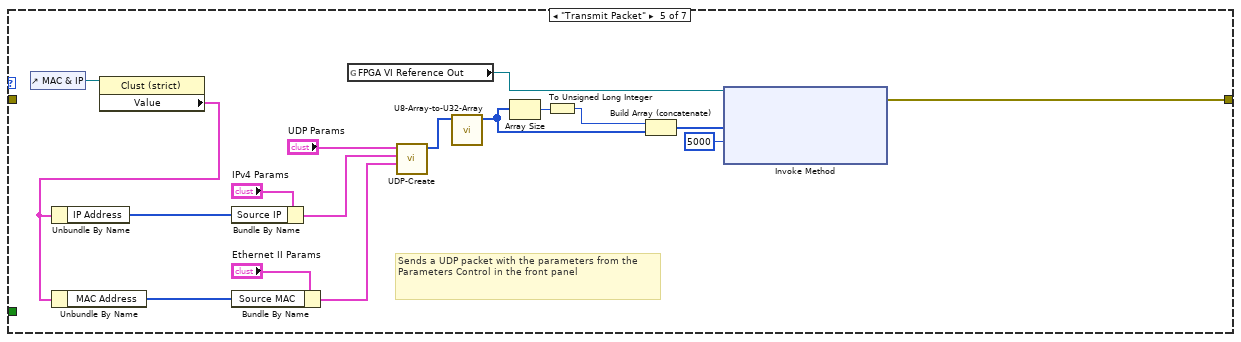
[diagram p8: hidden frame]
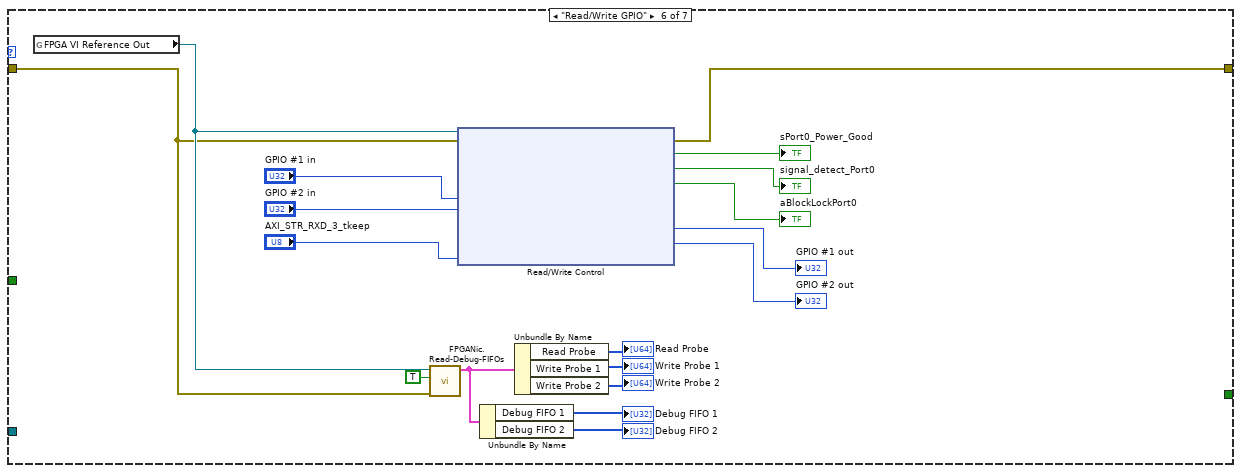
[diagram p9: hidden frame]
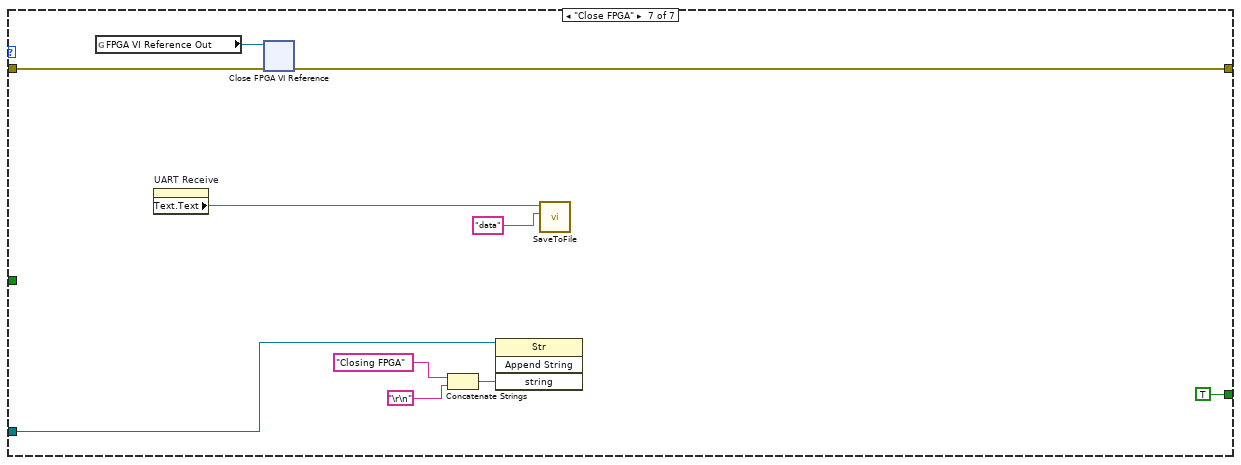
[diagram p10: hidden frame]
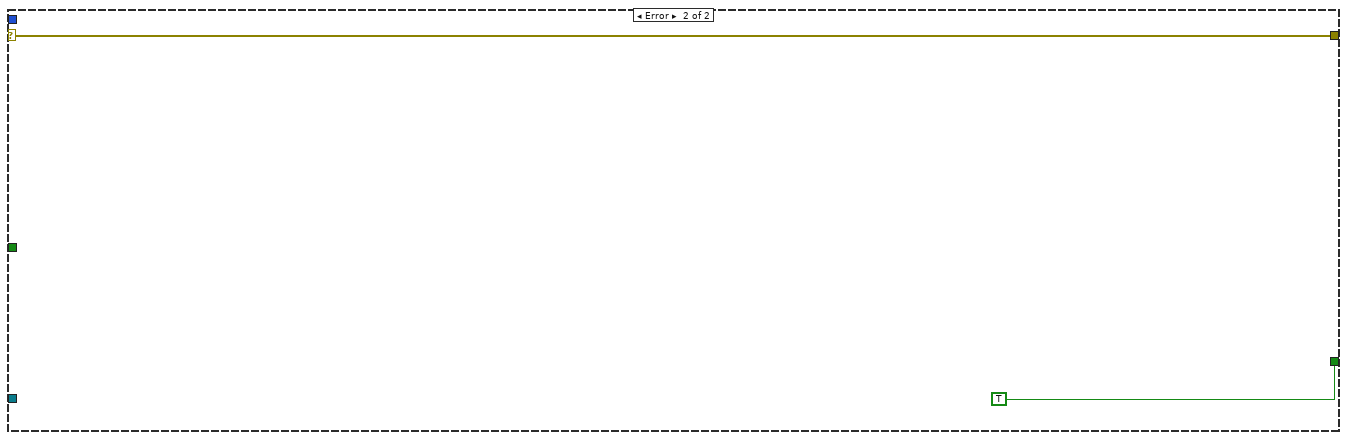
[diagram p11: hidden frame]
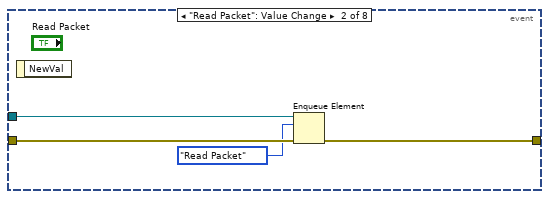
[diagram p14: hidden frame]
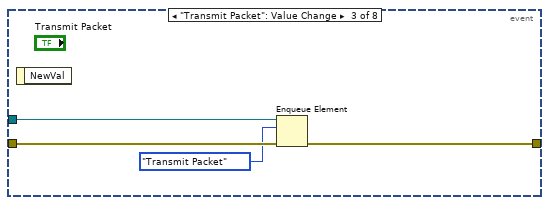
[diagram p15: hidden frame]
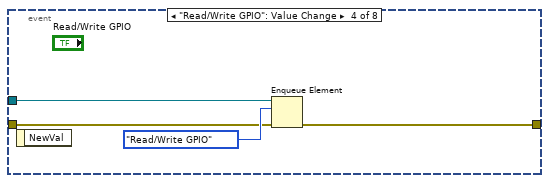
[diagram p16: hidden frame]
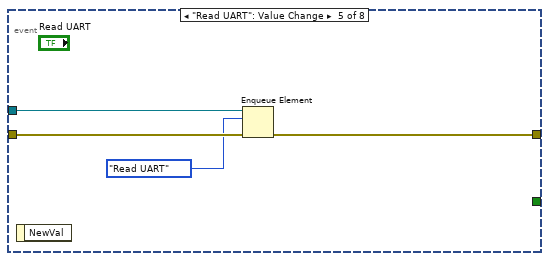
[diagram p17: hidden frame]
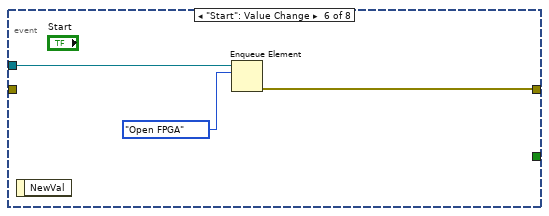
[diagram p18: hidden frame]
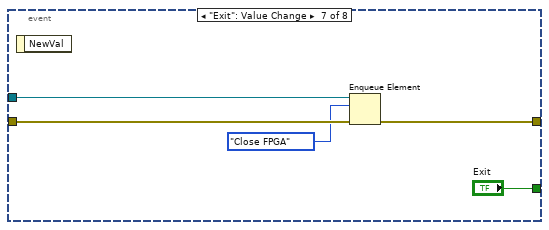
[diagram p19: hidden frame]
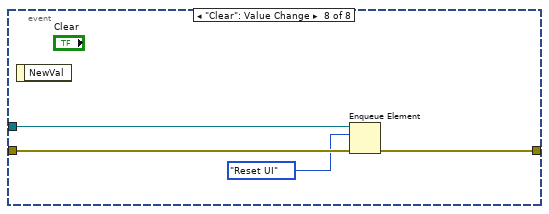
[diagram p20: hidden frame]
diagram:
  n1 = call <vilib>:"Application Directory.vi"() -> ("Application Directory"=w4:path)
  n2 = control-ref of="Clear Debug FIFOS?"() -> (w8:refnum<vi>)
  n3 = control-ref of="Status"() -> (w9:refnum<vi>)
  n4 = Obtain Queue(element data type=FPGANic.Events."Open FPGA" ("Enum"), error in (no error)="error in") -> (queue out=w1:refnum<queue>)  [unwired: 3 in, 2 out]
  n5 = call "Logging.Start.vi"("error in (no error)"="error in", "Root Folder"=w4) -> ("error out"=w6:errorcluster)  [unwired: 9 in]
  n6 = while {
    tunnel: w1 -> [w19]
    shift-right: [w14] -> w5
    shift-left: w6 -> [w15]
    tunnel: w9 -> [w13]
    tunnel: w8 -> [w12]
    stop <- w16 stop-if-true
    n7 = property class="Bool (strict)"(reference=w12) -> ("Value"=w11:bool)  [unwired: 1 in, 2 out]
    n8 = Dequeue Element(queue=w19, error in (no error)=w15) -> (element=w17:T6, error out=w18:errorcluster)  [unwired: 1 in, 2 out]
    n9 = case shown="No Error" w18 {
      selector: w18 -> [w20 w180]
      tunnel: w17 -> [w25 _]
      tunnel: [w24 TRUE] -> w16
      tunnel: [w23 w180] -> w14
      tunnel: w13 -> [w22 _]
      tunnel: w11 -> [w21 _]
      frame No Error {
        n10 = case shown="\"Read UART\"" w25 {
          tunnel: [_ _ _ _ _ _ TRUE] -> w24
          tunnel: [w27 w66 w101 w102 w149 w161 w178] -> w23
          tunnel: w22 -> [w49 w62 _ _ _ _ w174]
          tunnel: w21 -> [_ w64 _ w104 _ _ _]
          tunnel: w20 -> [w34 _ _ w105 _ w153 w172]
          frame "Open FPGA", Default {
            n11 = call <vilib>:"Info.vi"("Error In"=w34, "Message"="Opening FPGA") -> ("Error Out"=w33:errorcluster)  [unwired: 9 in]
            n12 = Open Dynamic Bitfile Reference(0:"Device address", 1:"lvbitx file", 2:TRUE ("Run When Loaded"), 3:w33, 4:refnum<k20> refnum ("FPGA VI Reference Out")) -> (5:w43:refnum<k20>, 8:w42:errorcluster)
            n13 = flat-sequence {
              tunnel: w43 -> [w61]
              tunnel: w42 -> [w60]
              tunnel: [w59] -> w39
              tunnel: [w58] -> w31
              tunnel: [TRUE] -> w38
              frame #0 {
                n14 = xnode "Invoke Method"("FPGA VI Reference In"=w61, "error in"=w60) -> ("FPGA VI Reference Out"=w59:refnum<k20>, "error out"=w58:errorcluster)
              }
            }
            n15 = invoke class="Str" method="Reinit To Default"(reference=w49) -> (reference out=w48:refnum<vi>)  [unwired: 2 in, 2 out]
            n16 = call <vilib>:"Info.vi"("Error In"=w31, "Message"="Bitstream Downloaded") -> ("Error Out"=w30:errorcluster)  [unwired: 9 in]
            n17 = xnode "Read/Write Control"("FPGA VI Reference In"=w39, "error in"=w30, "d_microblaze_i\\reset_rtl"=TRUE ("d_microblaze_i\\reset_rtl")) -> ("FPGA VI Reference Out"=w41:refnum<k20>, "error out"=w40:errorcluster)
            n18 = Concatenate Strings("Opening FPGA" ("string"), "\r\n") -> (w52:string)
            n19 = invoke class="Str" method="Append String"(reference=w48, "string"=w52) -> ()  [unwired: 2 in, 4 out]
            n20 = xnode "Invoke Method"("FPGA VI Reference In"=w41, "error in"=w40) -> ("FPGA VI Reference Out"=w36:refnum<k20>, "error out"=w28:errorcluster)  [unwired: 1 in]
            n21 = case shown="Error" w28 {
              tunnel: [TRUE FALSE] -> w35
              tunnel: ["FPGA Running" ("Message") "FPGA Not Running" ("Message")] -> w26
              frame No Error {
              }
              frame Error {
              }
            }
            "FPGA Ready" <- w35
            n22 = global write "FPGANic.Globals.vi" "FPGA VI Reference Out"(w36) -> ()
            n23 = call <vilib>:"Info.vi"("Error In"=w28, "Message"=w26) -> ("Error Out"=w27:errorcluster)  [unwired: 9 in]
            "Bitfile Downloaded" <- w38
          }
          frame "Read Packet" {
            n24 = global read "FPGANic.Globals.vi" "FPGA VI Reference Out"() -> (w63:refnum<k20>)
            n25 = xnode "Invoke Method"("FPGA VI Reference In"=w63, "Number of Elements"=u32 0, "Timeout (ms)"=250) -> ("FPGA VI Reference Out"=w68:refnum<k20>, "error out"=w67:errorcluster, "Elements Remaining"=w65:u32)  [unwired: 1 in, 1 out]
            n26 = Greater Than 0?(x=w65) -> (x > 0?=w69:bool)
            n27 = case shown="True" w69 {
              tunnel: w68 -> [_ w86]
              tunnel: w67 -> [w72 w85]
              tunnel: [w72 w83] -> w66
              tunnel: w65 -> [_ w84]
              tunnel: w64 -> [_ _]
              tunnel: w62 -> [_ w77]
              frame False {
              }
              frame True {
                # "Responds to\nARP and ICMP (ping)"
                # "Process incoming\nframes, get array\nof response frames"
                n28 = control-ref of="MAC & IP"() -> (w80:refnum<vi>)
                n29 = xnode "Invoke Method"("FPGA VI Reference In"=w86, "error in"=w85, "Number of Elements"=w84, "Timeout (ms)"=5000) -> ("FPGA VI Reference Out"=w78:refnum<k20>, "error out"=w83:errorcluster, "Data"=w82:u64[])  [unwired: 1 out]
                n30 = property class="Clust (strict)"(reference=w80) -> ("Value"=w79:T5)  [unwired: 1 in, 2 out]
                n31 = call <vilib>:"Info.vi"("Message"="DATA READ!") -> ("Error Out"=w73:errorcluster)  [unwired: 10 in]
                n32 = call "Process-Ethernet-Frames.vi"("Source Machine\nSettings"=w79, "Raw Data\nStream"=w82) -> ("UDP Payload"=→"In Payload":u8[], "Messages"=w76:string[], "Frames to send"=w81:u8[][])  [unwired: 7 in]
                n33 = for {
                  tunnel: w81 -> [w100] mode=indexing
                  tunnel: w78 -> [w94]
                  # "Prepend\nframe size\nin words"
                  # "Sending\nto FPGA\nfor Transmission"
                  # "Convert frame\nto U32"
                  n34 = call "U8-Array-to-U32-Array.vi"("Frame U8[] in"=w100) -> ("Frame U32[] out"=w95:u32[])  [unwired: 10 in]
                  n35 = Array Size(array=w95) -> (size(s)=w99:i32)
                  n36 = To Unsigned Quad Integer(1:w99) -> (0:w98:u64)
                  n37 = Build Array (concatenate)(w98, w95) -> (w97:u64[])
                  n38 = xnode "Invoke Method"("FPGA VI Reference In"=w94, "Data"=w97, "Timeout (ms)"=5000) -> ()  [unwired: 1 in, 3 out]
                }
                n39 = for {
                  tunnel: w77 -> [w91]
                  tunnel: w76 -> [w89] mode=indexing
                  shift-right: [w88] -> _
                  shift-left: w73 -> [w90]
                  n40 = Concatenate Strings(w89, "\r\n") -> (w93:string)
                  n41 = invoke class="Str" method="Append String"(reference=w91, error in=w90, "string"=w93) -> (error out=w88:errorcluster)  [unwired: 1 in, 3 out]
                  n42 = call <vilib>:"Info.vi"("Message"=w89) -> ()  [unwired: 10 in, 1 out]
                }
              }
            }
          }
          frame "Reset UI" {
            n43 = invoke class="VI" method="Default Vals.Reinit All"() -> (error out=w101:errorcluster)  [unwired: 3 in, 2 out]
          }
          frame "Read UART" {
            n44 = global read "FPGANic.Globals.vi" "FPGA VI Reference Out"() -> (w106:refnum<k20>)
            n45 = xnode "Invoke Method"("FPGA VI Reference In"=w106, "error in"=w105, "Number of Elements"=u32 0, "Timeout (ms)"=250) -> ("FPGA VI Reference Out"=w113:refnum<k20>, "error out"=w112:errorcluster, "Elements Remaining"=w109:u32)  [unwired: 1 out]
            n46 = Greater Than 0?(x=w109) -> (x > 0?=w111:bool)
            n47 = property on="UART Receive" class="Str"("Text.Scroll Position"=u32 999999) -> ()  [unwired: 2 in, 2 out]
            n48 = feedback #1("") -> (w110:string)
            n49 = case shown="True" w111 {
              tunnel: w110 -> [w118 w134]
              tunnel: w109 -> [_ w133]
              tunnel: w112 -> [w117 w131]
              tunnel: w113 -> [w116 w130]
              tunnel: [w118 w126] -> w107
              tunnel: [w117 w121] -> w102
              tunnel: w104 -> [_ w128]
              tunnel: [w116 w124] -> _
              frame False {
              }
              frame True {
                n50 = xnode "Invoke Method"("FPGA VI Reference In"=w130, "error in"=w131, "Number of Elements"=w133, "Timeout (ms)"=5000) -> ("FPGA VI Reference Out"=w124:refnum<k20>, "error out"=w122:errorcluster, "Data"=w125:u8[])  [unwired: 1 out]
                n51 = Type Cast(type="", x=w125) -> (*(type *) &x=w123:string)
                n52 = Concatenate Strings(w134, w123) -> (w129:string)
                n53 = Concatenate Strings("UART: " ("string"), w123) -> (w120:string)
                n54 = Select(t=w123, s=w128, f=w129) -> (s? t:f=w126:string)
                n55 = call <vilib>:"Info.vi"("Error In"=w122, "Message"=w120) -> ("Error Out"=w121:errorcluster)  [unwired: 9 in]
              }
            }
            "UART Receive" <- w107
            n56 = feedback-in #1(w107) -> ()
          }
          frame "Transmit Packet" {
            # "Sends a UDP packet with the parameters from the\nParameters Control in the front panel"
            n57 = control-ref of="MAC & IP"() -> (w138:refnum<vi>)
            n58 = property class="Clust (strict)"(reference=w138) -> ("Value"=w136:T5)  [unwired: 1 in, 2 out]
            n59 = Unbundle By Name(w136) -> ("IP Address"=w137:u8[])
            n60 = Unbundle By Name(w136) -> ("MAC Address"=w135:u8[])
            n61 = Bundle By Name(cluster="IPv4 Params", "Source IP"=w137) -> (w139:T3)
            n62 = Bundle By Name(cluster="Ethernet II Params", "Source MAC"=w135) -> (w140:T2)
            n63 = global read "FPGANic.Globals.vi" "FPGA VI Reference Out"() -> (w148:refnum<k20>)
            n64 = call "UDP-Create.vi"("Ethernet II Params"=w140, "IPv4 Params"=w139, "UDP Params"="UDP Params") -> ("Ethernet Frame"=w147:u8[])  [unwired: 6 in, 2 out]
            n65 = call "U8-Array-to-U32-Array.vi"("Frame U8[] in"=w147) -> ("Frame U32[] out"=w144:u32[])  [unwired: 10 in]
            n66 = Array Size(array=w144) -> (size(s)=w146:i32)
            n67 = To Unsigned Long Integer(number=w146) -> (unsigned 32bit integer=w145:u32)
            n68 = Build Array (concatenate)(w145, w144) -> (w143:u32[])
            n69 = xnode "Invoke Method"("FPGA VI Reference In"=w148, "Data"=w143, "Timeout (ms)"=5000) -> ("error out"=w149:errorcluster)  [unwired: 1 in, 2 out]
          }
          frame "Read/Write GPIO" {
            n70 = global read "FPGANic.Globals.vi" "FPGA VI Reference Out"() -> (w154:refnum<k20>)
            n71 = call "FPGANic.Read-Debug-FIFOs.vi"("error in"=w153, "Clear Debug FIFOs"=TRUE, "FPGA VI Reference In"=w154) -> ("Debug Data"=w159:T7)  [unwired: 7 in, 1 out]
            n72 = xnode "Read/Write Control"("FPGA VI Reference In"=w154, "error in"=w153, "GPIO #1 in"="GPIO #1 in", "GPIO #2 in"="GPIO #2 in", "d_microblaze_i\\AXI_STR_RXD_3_tkeep"="AXI_STR_RXD_3_tkeep") -> ("error out"=w161:errorcluster, "sPort0_Power_Good"=→"sPort0_Power_Good":bool, "signal_detect_Port0"=→"signal_detect_Port0":bool, "aBlockLockPort0"=→"aBlockLockPort0":bool, "GPIO #1 out"=→"GPIO #1 out":u32, "GPIO #2 out"=→"GPIO #2 out":u32)  [unwired: 1 out]
            n73 = Unbundle By Name(w159) -> ("Debug FIFO 1"=→"Debug FIFO 1":u32[], "Debug FIFO 2"=→"Debug FIFO 2":u32[])
            n74 = Unbundle By Name(w159) -> ("Read Probe"=→"Read Probe":u64[], "Write Probe 1"=→"Write Probe 1":u64[], "Write Probe 2"=→"Write Probe 2":u64[])
          }
          frame "Close FPGA" {
            n75 = global read "FPGANic.Globals.vi" "FPGA VI Reference Out"() -> (w173:refnum<k20>)
            n76 = property on="UART Receive" class="Str"() -> ("Text.Text"=w171:string)  [unwired: 2 in, 2 out]
            n77 = xnode "Close FPGA VI Reference"("FPGA VI Reference In"=w173, "error in"=w172) -> ("error out"=w178:errorcluster)
            n78 = Concatenate Strings("Closing FPGA" ("string"), "\r\n") -> (w177:string)
            n79 = invoke class="Str" method="Append String"(reference=w174, "string"=w177) -> ()  [unwired: 2 in, 4 out]
            n80 = call "SaveToFile.vi"("FileNamePrefix"="data" ("Text.Text"), "TextToWrite"=w171) -> ()  [unwired: 10 in]
          }
        }
      }
      frame Error {
      }
    }
    "error out" <- w14
  }
  n81 = Enqueue Element(queue=w1, element=FPGANic.Events."Open FPGA" ("Enum")) -> ()  [unwired: 2 in, 3 out]
  n82 = while {
    tunnel: w1 -> [w188]
    shift-right: [w183] -> w10
    shift-left: _ -> [w184]
    stop <- w186 stop-if-true
    n83 = event shown="[0] Timeout" {
      selector: _ -> [_ _ _ _ _ _ _ _]
      dyn-events: _ -> [_ _ _ _ _ _ _ _]
      timeout: 50 -> [_ _ _ _ _ _ _ _]
      tunnel: w188 -> [w190 w202 w206 w209 w214 w216 w222 w226]
      tunnel: [_ w201 w204 w207 w211 w215 w221 w225] -> w183
      tunnel: [_ _ _ _ _ _ "Exit" _] -> w185
      tunnel: w184 -> [w189 w200 w205 w208 w213 _ w219 w224]
      event Timeout {
        n84 = event-data() -> ()  [unwired: 1 in, 3 out]
        n85 = case shown="True" "UART Polling?" {
          tunnel: w190 -> [_ w197]
          tunnel: w189 -> [_ w196]
          frame False {
          }
          frame True {
            n86 = Enqueue Element(queue=w197, element=FPGANic.Events."Read UART" ("Enum"), error in (no error)=w196) -> ()  [unwired: 1 in, 3 out]
          }
        }
        n87 = case shown="True" "Read Polling?" {
          tunnel: w190 -> [_ w194]
          tunnel: w189 -> [_ w193]
          frame False {
          }
          frame True {
            n88 = Enqueue Element(queue=w194, element=FPGANic.Events."Read Packet" ("Enum"), error in (no error)=w193) -> ()  [unwired: 1 in, 3 out]
          }
        }
      }
      event "Read Packet": Value Change {
        n89 = event-data() -> ()  [unwired: 1 in, 1 out]
        n90 = Enqueue Element(queue=w202, element=FPGANic.Events."Read Packet" ("Enum"), error in (no error)=w200) -> (error out=w201:errorcluster)  [unwired: 1 in, 2 out]
      }
      event "Transmit Packet": Value Change {
        n91 = event-data() -> ()  [unwired: 1 in, 1 out]
        n92 = Enqueue Element(queue=w206, element=FPGANic.Events."Transmit Packet" ("Enum"), error in (no error)=w205) -> (error out=w204:errorcluster)  [unwired: 1 in, 2 out]
      }
      event "Read/Write GPIO": Value Change {
        n93 = event-data() -> ()  [unwired: 1 in, 1 out]
        n94 = Enqueue Element(queue=w209, element=FPGANic.Events."Read/Write GPIO" ("Enum"), error in (no error)=w208) -> (error out=w207:errorcluster)  [unwired: 1 in, 2 out]
      }
      event "Read UART": Value Change {
        n95 = event-data() -> ()  [unwired: 1 in, 1 out]
        n96 = Enqueue Element(queue=w214, element=FPGANic.Events."Read UART" ("Enum"), error in (no error)=w213) -> (error out=w211:errorcluster)  [unwired: 1 in, 2 out]
      }
      event "Start": Value Change {
        n97 = event-data() -> ()  [unwired: 1 in, 1 out]
        n98 = Enqueue Element(queue=w216, element=FPGANic.Events."Open FPGA" ("Enum")) -> (error out=w215:errorcluster)  [unwired: 2 in, 2 out]
      }
      event "Exit": Value Change {
        n99 = event-data() -> ()  [unwired: 1 in, 1 out]
        n100 = Enqueue Element(queue=w222, element=FPGANic.Events."Close FPGA" ("Enum"), error in (no error)=w219) -> (error out=w221:errorcluster)  [unwired: 1 in, 2 out]
      }
      event "Clear": Value Change {
        n101 = event-data() -> ()  [unwired: 1 in, 1 out]
        n102 = Enqueue Element(queue=w226, element=FPGANic.Events."Reset UI" ("Enum"), error in (no error)=w224) -> (error out=w225:errorcluster)  [unwired: 1 in, 2 out]
      }
    }
    n103 = Unbundle By Name(w183) -> ("status"=w187:bool)
    n104 = Or(x=w187, y=w185) -> (x .or. y?=w186:bool)
  }
  n105 = Release Queue(queue=w1, error in (no error)=w10) -> ()  [unwired: 1 in, 3 out]
  n106 = call "Logging.Stop.vi"("error in (no error)"=w5) -> ()  [unwired: 10 in, 1 out]
